vi "Get Key Path.vi"(7 "rel_path":string, 8 "error in (no error)":errorcluster, 9 "default value":path, 10 "key":string, 11 "section":string) -> (0 "error out":errorcluster, 3 "value":path)   [LabVIEW 2016]
uses:
  <vilib>/Utility/config.llb/Read Key (Path).vi
  <vilib>/Utility/config.llb/NI_LVConfig.lvlib
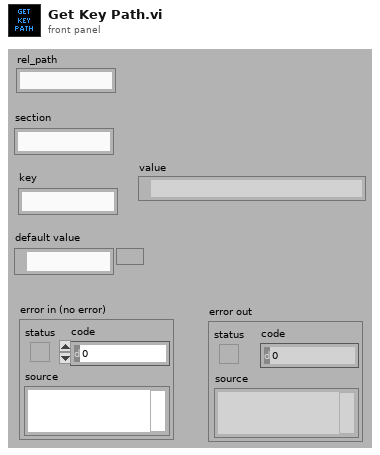
[diagram p1: front panel]
types:
  T1 = enum32{"invalid app kind", "Development System", "Run Time System", "Student Edition", "Embedded LabVIEW", "Evaluation", "Custom"}
  T2 = typedef "NI_LVConfig.lvlib/Config Data RefNum.ctl" = refnum<k1>
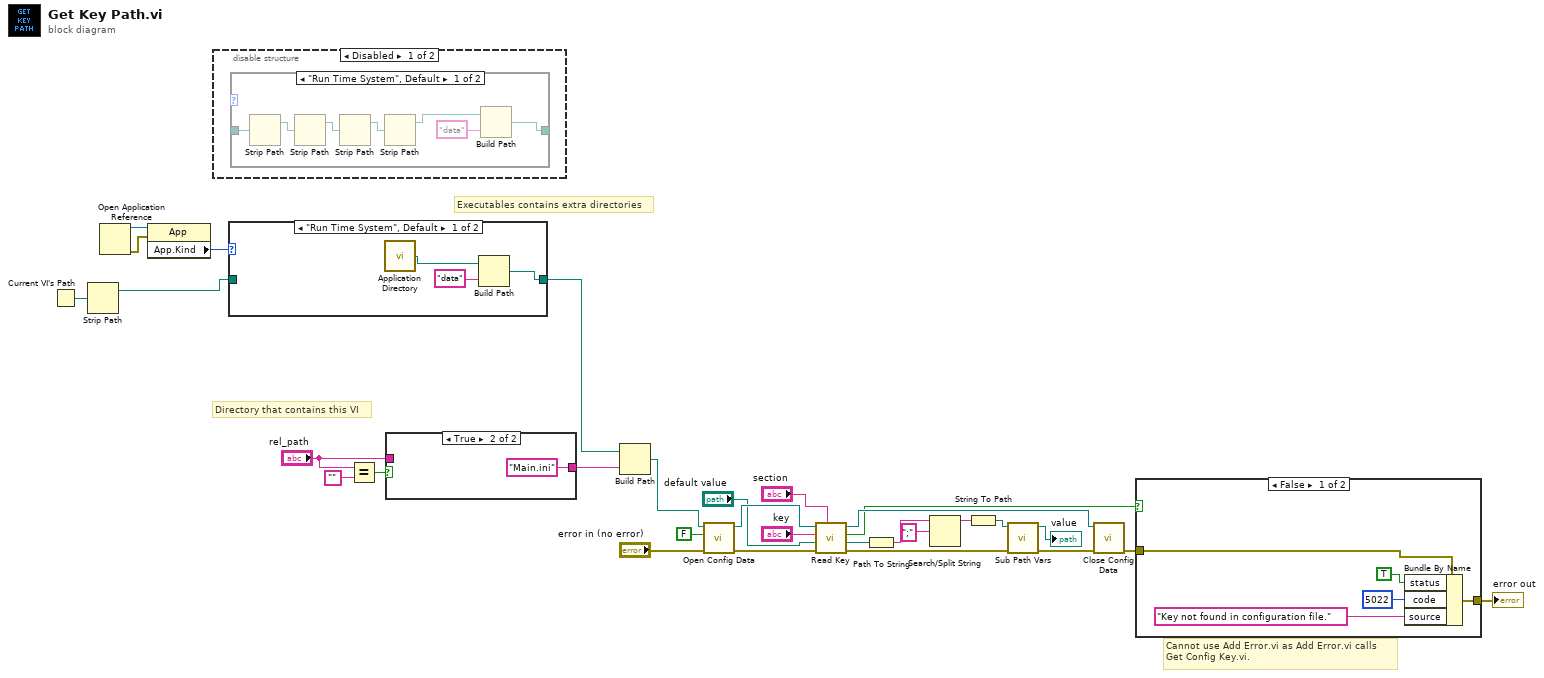
[diagram p0: block diagram]
diagram:
  # "Executables contains extra directories"
  # "Directory that contains this VI"
  # "Cannot use Add Error.vi as Add Error.vi calls\nGet Config Key.vi."
  n1 = Current VI's Path() -> (path=w6:path)
  n2 = Strip Path(path=w6) -> (stripped path=w3:path)  [unwired: 1 out]
  n3 = Open Application Reference() -> (0:w4:errorcluster, 3:w5:refnum<vi>)  [unwired: 4 in]
  n4 = property class="App"(reference=w5, error in=w4) -> ("App.Kind"=w2:T1)  [unwired: 2 out]
  n5 = disable-structure shown="Disabled" {
    frame Disabled {
      n6 = case shown="\"Run Time System\", Default" {
        selector: _ -> [_ _]
        tunnel: _ -> [w31 w38]
        tunnel: [w36 w38] -> _
        frame "Run Time System", Default {
          n7 = Strip Path(path=w31) -> (stripped path=w33:path)  [unwired: 1 out]
          n8 = Strip Path(path=w33) -> (stripped path=w32:path)  [unwired: 1 out]
          n9 = Strip Path(path=w32) -> (stripped path=w37:path)  [unwired: 1 out]
          n10 = Strip Path(path=w37) -> (stripped path=w35:path)  [unwired: 1 out]
          n11 = Build Path(base path=w35, name or relative path="data") -> (appended path=w36:path)
        }
        frame "Development System" {
        }
      }
    }
    frame Enabled {
    }
  }
  n12 = case shown="\"Run Time System\", Default" w2 {
    tunnel: w3 -> [_ w42]
    tunnel: [w41 w42] -> w1
    frame "Run Time System", Default {
      n13 = call <vilib>:"Application Directory.vi"() -> ("Application Directory"=w39:path)
      n14 = Build Path(base path=w39, name or relative path="data") -> (appended path=w41:path)
    }
    frame "Development System" {
    }
  }
  n15 = Equal?(x="rel_path", y="") -> (x = y?=w12:bool)
  n16 = case shown="True" w12 {
    tunnel: [w43 "Main.ini" ("name or relative path")] -> w10
    tunnel: "rel_path" -> [w43 _]
    frame False {
    }
    frame True {
    }
  }
  n17 = Build Path(base path=w1, name or relative path=w10) -> (appended path=w30:path)
  n18 = call <vilib>:"Open Config Data.vi"("error in (no error)"="error in (no error)", "create file if necessary (T)"=FALSE, "configuration file path"=w30) -> ("error out"=w25:errorcluster, "refnum"=w28:T2)  [unwired: 6 in, 1 out]
  n19 = call-poly <vilib>:"Read Key.vi"("section"="section", "error in (no error)"=w25, "default value"="default value", "key"="key", "refnum"=w28) -> ("error out"=w14:errorcluster, "value"=w15:path, "found?"=w7:bool, "refnum out"=w24:T2)  [unwired: 3 in]
  n20 = Path To String(path=w15) -> (string=w19:string)
  n21 = Search/Split String(string=w19, search string/char (-)=";") -> (substring before match=w17:string)  [unwired: 1 in, 2 out]
  n22 = String To Path(string=w17) -> (path=w16:path)
  n23 = call "Sub Path Vars.vi"("error in (no error)"=w14, "path"=w16) -> ("error out"=w20:errorcluster, "abs path"=→"value":path)  [unwired: 8 in]
  n24 = call <vilib>:"Close Config Data.vi"("error in (no error)"=w20, "refnum"=w24) -> ("error out"=w8:errorcluster)  [unwired: 8 in, 1 out]
  n25 = case shown="False" w7 {
    tunnel: [w47 w50] -> w9
    tunnel: w8 -> [w45 w50]
    frame False {
      n26 = Bundle By Name(cluster=w45, "status"=TRUE, "code"=5022, "source"="Key not found in configuration file.") -> (w47:errorcluster)
    }
    frame True {
    }
  }
  "error out" <- w9
